vi "addBinaryElement.vi"(6 "Type":T1 items=["Generic"=0, "Function"=1, "Binary (Old)"=2, "UUID"=3, "MD5"=5, "User Defined"=128], 7 "Name":string, 8 "error in (no error)":errorcluster, 9 "Value":u8[](array[numeric]), 10 "Replace? (false)":bool, 11 "tBSONDocument in":refnum<class "tBSONDocument.lvclass">) -> (0 "error out":errorcluster, 3 "tBSONDocument out":refnum<class "tBSONDocument.lvclass">)   [LabVIEW 2013, in "BSON.lvlib" / "tBSONDocument.lvclass"]
doc: "Adds a binary blob (an array of U8s) to a BSON document."
uses:
  tBSONDocument.lvclass
  BSONElements/tBSONBinary/Subtype.ctl
  BSONElements/tBSONBinary/tBSONBinary.lvclass
  tBSONElement/tBSONElement.lvclass
  tBSONElement/setName.vi
  BSONElements/tBSONBinary/setSubtype.vi
  BSONElements/tBSONBinary/setValue.vi
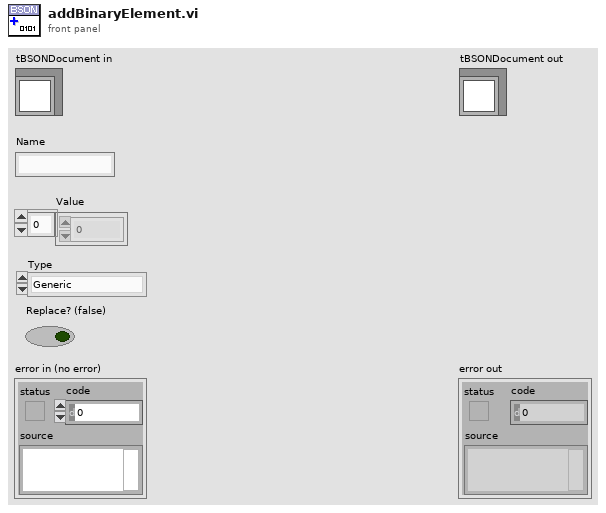
[diagram p1: front panel]
types:
  T1 = typedef "BSON.lvlib/tBSONBinary.lvclass/Subtype.ctl" = u8
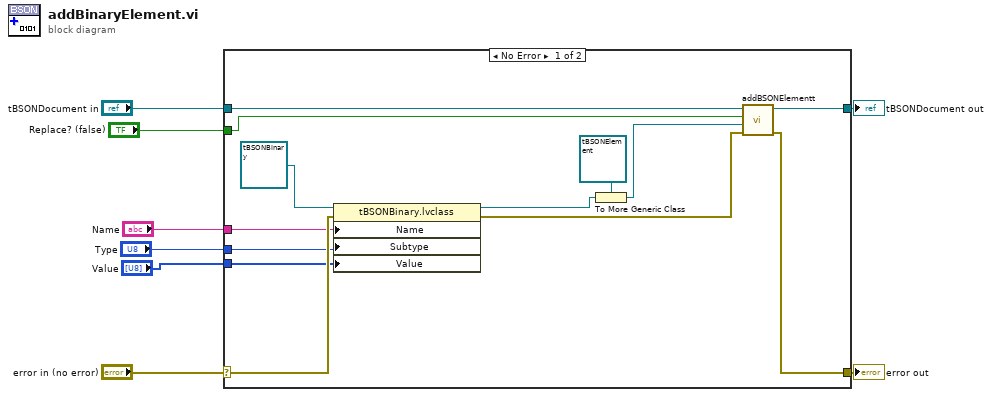
[diagram p0: block diagram]
diagram:
  n1 = case shown="No Error" "error in (no error)" {
    selector: "error in (no error)" -> [w18 w23]
    tunnel: [w16 w23] -> w7
    tunnel: [w21 w22] -> w5
    tunnel: "tBSONDocument in" -> [w20 w22]
    tunnel: "Name" -> [w12 _]
    tunnel: "Type" -> [w11 _]
    tunnel: "Value" -> [w10 _]
    tunnel: "Replace? (false)" -> [w9 _]
    frame No Error {
      n2 = property class="tBSONBinary.lvclass"(reference=refnum<class "tBSONBinary.lvclass"> refnum ("BSON.lvlib:tBSONBinary.lvclass"), error in=w18, "Name"=w12, "Subtype"=w11, "Value"=w10) -> (reference out=w14:refnum<class "tBSONBinary.lvclass">, error out=w17:errorcluster)
      n3 = To More Generic Class(target class=refnum<class "tBSONElement.lvclass"> refnum ("BSON.lvlib:tBSONElement.lvclass"), reference=w14) -> (generic class reference=w13:refnum<class "tBSONElement.lvclass">)
      n4 = call "addBSONElementt.vi"("error in (no error)"=w17, "Element"=w13, "Replace? (false)"=w9, "tBSONDocument in"=w20) -> ("error out"=w16:errorcluster, "tBSONDocument out"=w21:refnum<class "tBSONDocument.lvclass">)  [unwired: 6 in]
    }
    frame Error {
    }
  }
  "error out" <- w7
  "tBSONDocument out" <- w5
